vi "Labbyy Bird.vi"() -> ()   [LabVIEW 2014]
uses:
  <vilib>/Utility/miscctls.llb/LVPointTypeDef.ctl
  Labby Bird/Labby Bird/Labby bird-Support.llb/Prune below.vi
  Labby Bird/Labby Bird/Labby bird-Support.llb/Global-1.vi
  <vilib>/Utility/inputDevices.llb/mouseAcquire.vi
  Labby Bird/Labby Bird/Labby bird-Support.llb/Generate rand. pipe locations.vi
  <vilib>/Utility/inputDevices.llb/closeMouse.vi
  <vilib>/Analysis/NI_AALBase.lvlib
panel:
  out "SCORE":dbl
  in  "UP":bool
  out "XY Graph":cluster{dbl[], dbl[]}[](graph)
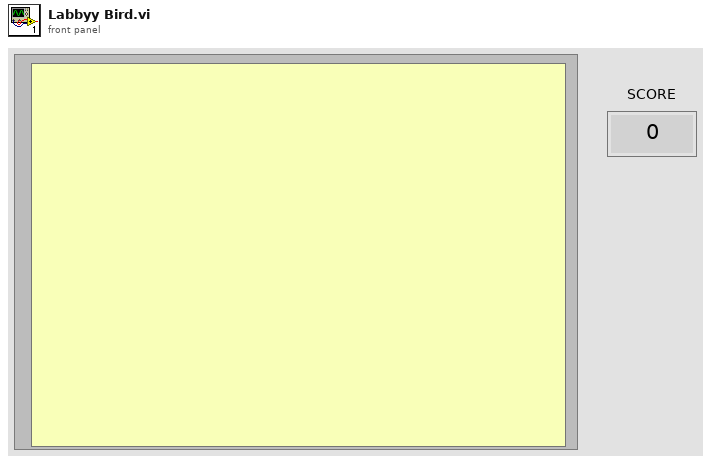
[diagram p1: front panel]
types:
  T1 = typedef "LVPointTypeDef.ctl" = cluster{"Horizontal":i16, "Vertical":i16}
  T2 = cluster{"button 1":bool, "button 2":bool, "button 3":bool, "button 4":bool}
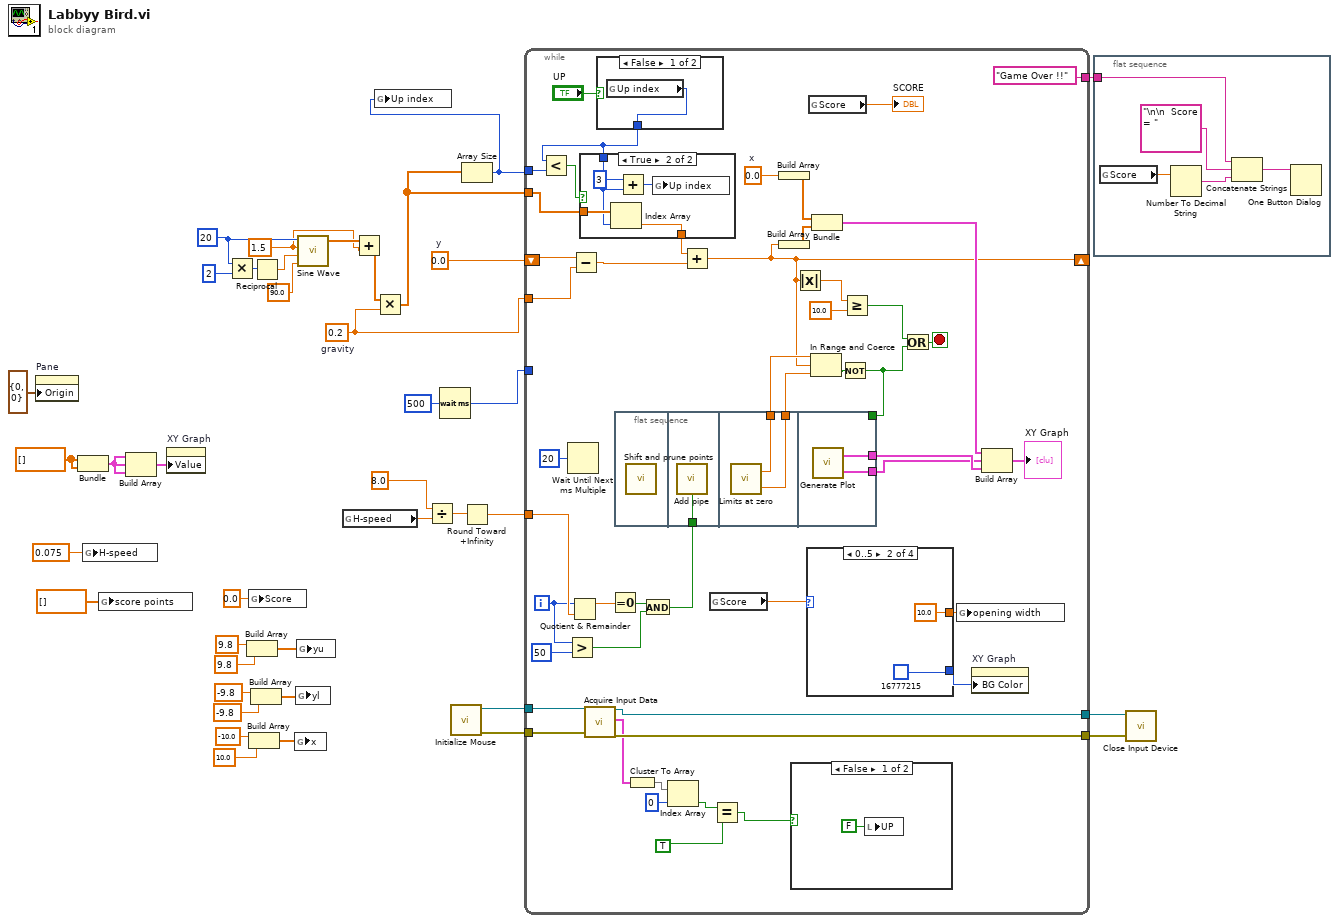
[diagram p0: block diagram]
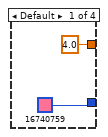
[diagram p2: hidden frame]
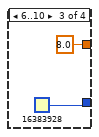
[diagram p3: hidden frame]
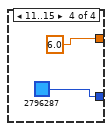
[diagram p4: hidden frame]
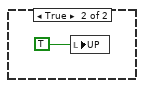
[diagram p5: hidden frame]
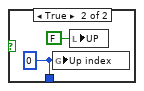
[diagram p6: hidden frame]
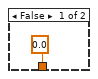
[diagram p7: hidden frame]
diagram:
  w14 = dbl[] []
  w29 = 1.5 ("amplitude")
  w37 = 20 ("samples")
  w31 = 0.2  # gravity
  w39 = 0.0  # y
  n1 = property on="Pane" class="Pane"("Origin"=T1 {"Horizontal"=0, "Vertical"=0}) -> ()  [unwired: 2 in, 2 out]
  n2 = Bundle(w14, w14) -> (w15:cluster{dbl[], dbl[]})  [unwired: 1 in]
  n3 = global write "Global-1.vi" "H-speed"(0.075 ("H-speed")) -> ()
  n4 = global write "Global-1.vi" "score points"(dbl[] []) -> ()
  n5 = Build Array(w15, w15, w15) -> (w28:cluster{dbl[], dbl[]}[])
  n6 = property on="XY Graph" class="XYGraph (strict)"("Value"=w28) -> ()  [unwired: 2 in, 2 out]
  n7 = Multiply(x=w37, y=2) -> (x*y=w35:i32)
  n8 = Build Array(9.8 ("element"), 9.8 ("element")) -> (w16:dbl[])
  n9 = global write "Global-1.vi" "Score"(0.0 ("Score")) -> ()
  n10 = Build Array(-10.0 ("element"), 10.0 ("element")) -> (w18:dbl[])
  n11 = Build Array(-9.8 ("element"), -9.8 ("element")) -> (w17:dbl[])
  n12 = Reciprocal(x=w35) -> (1/x=w34:dbl)
  n13 = global write "Global-1.vi" "x"(w18) -> ()
  n14 = global write "Global-1.vi" "yl"(w17) -> ()
  n15 = global write "Global-1.vi" "yu"(w16) -> ()
  n16 = call <vilib>:"Sine Wave.vi"("samples"=w37, "amplitude"=w29, "frequency"=w34, "phase in"=90.0) -> ("sine wave"=w33:dbl[])  [unwired: 1 in, 2 out]
  n17 = global read "Global-1.vi" "H-speed"() -> (w12:dbl)
  n18 = Add(x=w33, y=w29) -> (x+y=w32:dbl[])
  n19 = Multiply(x=w32, y=w31) -> (x*y=w30:dbl[])
  n20 = Divide(x=8.0, y=w12) -> (x/y=w10:dbl)
  n21 = Wait (ms)(milliseconds to wait=u32 500) -> (millisecond timer value=w26:u32)
  n22 = call <vilib>:"Initialize Mouse.vi"() -> ("error out"=w4:errorcluster, "device ID"=w5:refnum<k1>)  [unwired: 10 in]
  n23 = Array Size(array=w30) -> (size(s)=w19:i32)
  n24 = global write "Global-1.vi" "Up index"(w19) -> ()
  n25 = Round Toward +Infinity(x=w10) -> (ceil(x): smallest int >= x=w9:dbl)
  n26 = while {
    tunnel: w31 -> [w80]
    shift-right: [w67] -> _
    shift-left: w39 -> [w81]
    tunnel: w30 -> [w77]
    tunnel: w19 -> [w79]
    tunnel: ["Game Over !!" ("message")] -> w8
    tunnel: w26 -> [_]
    tunnel: w9 -> [w61]
    tunnel: w5 -> [w52]
    tunnel: w4 -> [w51]
    tunnel: [w50] -> w3
    tunnel: [w49] -> w2
    i -> [w57]
    stop <- w53 stop-if-true
    w82 = 0.0  # x
    n27 = Greater?(x=w57, y=50) -> (0:w55:bool)
    n28 = Wait Until Next ms Multiple(millisecond multiple=u32 20) -> ()  [unwired: 1 out]
    n29 = Quotient & Remainder(x=w57, y=w61) -> (x-y*floor(x/y)=w60:dbl)  [unwired: 1 out]
    n30 = Subtract(x=w81, y=w80) -> (x-y=w76:dbl)
    n31 = call-poly <vilib>:"Acquire Input Data.vi"("device ID"=w52, "error in (no error)"=w51) -> ("device ID"=w49:refnum<k1>, "button info"=w48:T2, "error out"=w50:errorcluster)  [unwired: 14 in, 1 out]
    n32 = case shown="False" "UP" {
      tunnel: [w103 w104] -> w73
      frame False {
        n33 = global read "Global-1.vi" "Up index"() -> (w103:i32)
      }
      frame True {
        w104 = 0 ("Up index")
        n34 = global write "Global-1.vi" "Up index"(w104) -> ()
        n35 = local write "UP"(FALSE ("UP")) -> ()
      }
    }
    n36 = Less?(x=w73, y=w79) -> (x < y?=w78:bool)
    n37 = case shown="True" w78 {
      tunnel: w77 -> [_ w111]
      tunnel: w73 -> [_ w110]
      tunnel: [0.0 w109] -> w75
      frame False {
      }
      frame True {
        n38 = Index Array(array=w111, index=w110) -> (element=w109:dbl)
        n39 = Add(x=3, y=w110) -> (x+y=w108:i32)
        n40 = global write "Global-1.vi" "Up index"(w108) -> ()
      }
    }
    n41 = Equal To 0?(x=w60) -> (x = 0?=w59:bool)
    n42 = flat-sequence {
      tunnel: w58 -> [w98]
      tunnel: [w100] -> w69
      tunnel: [w99] -> w68
      tunnel: [w102] -> w64
      tunnel: [w101] -> w63
      tunnel: w62 -> [_]
      frame #0 {
        n43 = call "Shift and prune points.vi"() -> ()  [unwired: 12 in]
      }
      frame #1 {
        n44 = call "Add pipe.vi"("Add?"=w98) -> ()
      }
      frame #2 {
        n45 = call "Limits at zero.vi"() -> ("lower limit"=w99:dbl, "upper limit"=w100:dbl)  [unwired: 2 in]
      }
      frame #3 {
        n46 = call "Generate Plot.vi"() -> ("Lower"=w101:cluster{"x":dbl[], "yl":dbl[]}, "Upper"=w102:cluster{"x":dbl[], "yu":dbl[]})  [unwired: 2 in]
      }
    }
    n47 = Cluster To Array(cluster=w48) -> (array=w47:bool[])
    n48 = And(x=w59, y=w55) -> (x .and. y?=w58:bool)
    n49 = Index Array(array=w47, index=0) -> (element=w45:bool)
    n50 = Add(x=w75, y=w76) -> (x+y=w67:dbl)
    n51 = global read "Global-1.vi" "Score"() -> (w41:dbl)
    n52 = Equal?(x=w45, y=TRUE) -> (x = y?=w43:bool)
    n53 = Build Array(w82) -> (w84:dbl[])
    n54 = Build Array(w67) -> (w83:dbl[])
    n55 = case shown="False" w43 {
      frame False {
        n56 = local write "UP"(FALSE ("UP")) -> ()
      }
      frame True {
        n57 = local write "UP"(TRUE) -> ()
      }
    }
    n58 = Absolute Value(x=w67) -> (abs(x)=w85:dbl)
    n59 = case shown="0..5" w41 {
      tunnel: [u32 16740759 u32 16777215 u32 16383928 u32 2796287] -> w42
      tunnel: [4.0 ("opening width") 10.0 ("opening width") 8.0 ("opening width") 6.0 ("opening width")] -> w40
      frame Default {
      }
      frame 0..5 {
      }
      frame 6..10 {
      }
      frame 11..15 {
      }
    }
    n60 = global read "Global-1.vi" "Score"() -> (→"SCORE":dbl)
    n61 = In Range and Coerce(upper limit=w69, x=w67, lower limit=w68) -> (In Range?=w65:bool)  [unwired: 1 out]
    n62 = Bundle(w84, w83) -> (w72:cluster{dbl[], dbl[]})  [unwired: 1 in]
    n63 = Not(x=w65) -> (.not. x?=w62:bool)
    n64 = Greater Or Equal?(x=w85, y=10.0) -> (x >= y?=w66:bool)
    n65 = Or(x=w66, y=w62) -> (x .or. y?=w53:bool)
    n66 = global write "Global-1.vi" "opening width"(w40) -> ()
    n67 = property on="XY Graph" class="XYGraph (strict)"("BG Color"=w42) -> ()  [unwired: 2 in, 2 out]
    n68 = Build Array(w72, w63, w64) -> (→"XY Graph":cluster{"x":dbl[], "yu":dbl[]}[])
  }
  n69 = flat-sequence {
    tunnel: w8 -> [w112]
    frame #0 {
      n70 = global read "Global-1.vi" "Score"() -> (w116:dbl)
      n71 = Number To Decimal String(number=w116) -> (decimal integer string=w115:string)  [unwired: 1 in]
      n72 = Concatenate Strings(w112, "\n\n  Score = " ("string"), w115) -> (w113:string)
      n73 = One Button Dialog(message=w113) -> ()  [unwired: 1 in, 1 out]
    }
  }
  n74 = call-poly <vilib>:"Close Input Device.vi"("error in (no error)"=w3, "device ID"=w2) -> ()  [unwired: 8 in, 1 out]
